vi "main(test) (1).vi"() -> ()   [LabVIEW 2020]
uses:
  stany.ctl
  <vilib>/Analysis/1siggen.llb/Ramp Pattern by Samples.vi
  <vilib>/Utility/file.llb/Write Delimited Spreadsheet (DBL).vi
  lib/VirtualLab.lvlibp/VISASimulator/VISALib.lvlib
  <vilib>/Analysis/NI_AALBase.lvlib
panel:
  in  "save":bool
  out "Connection HP_dvm1":bool
  out "Actual Power [mW]":dbl
  in  "Pmax [mW]":dbl=200.0
  in  "Ib[uA]":dbl(ring) items=["0"=0.0, "100"=0.0001, "200"=0.0002, "300"=0.0003, "400"=0.0004]
  out "Ic=f(Uce)":cluster{dbl[], "Ramp Pattern":dbl[]}(graph)
  out "Ic[A]":dbl
  out "Uce [V]":dbl
  out "Uce=f(Upsu)":cluster{dbl[], "Ramp Pattern":dbl[]}(graph)
  in  "Cancel Button":bool
  out "Progres":u8(slide) scale=0.0..100.0
  in  "stop/resume":bool
  in  "Measure":bool
  in  "Connect":bool
  out "Connection HP_zas":bool
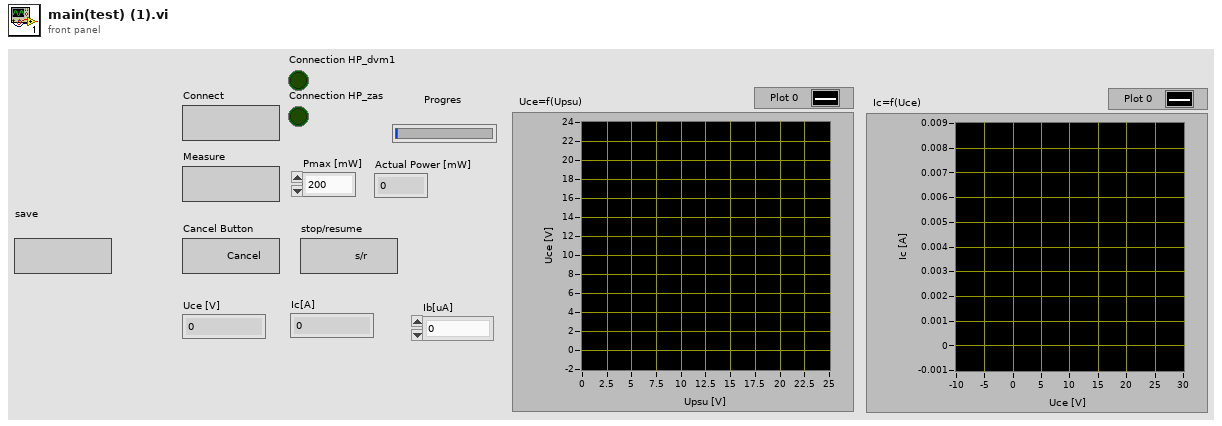
[diagram p1: front panel]
types:
  T1 = cluster{"connecton":bool, "HP_dvm1(DMM reference)":refnum<visa-resource-name>}
  T2 = cluster{"HP_zas (PSU reference)":refnum<visa-resource-name>, "connecton":bool, "Ic":dbl[], "Uce":dbl[]}
  T3 = typedef "stany.ctl" = enum16{"init", "wait", "connect", "measure", "end", "save", "error"}
  T4 = enum8{"Enabled", "Disabled", "Disabled and Grayed Out"}
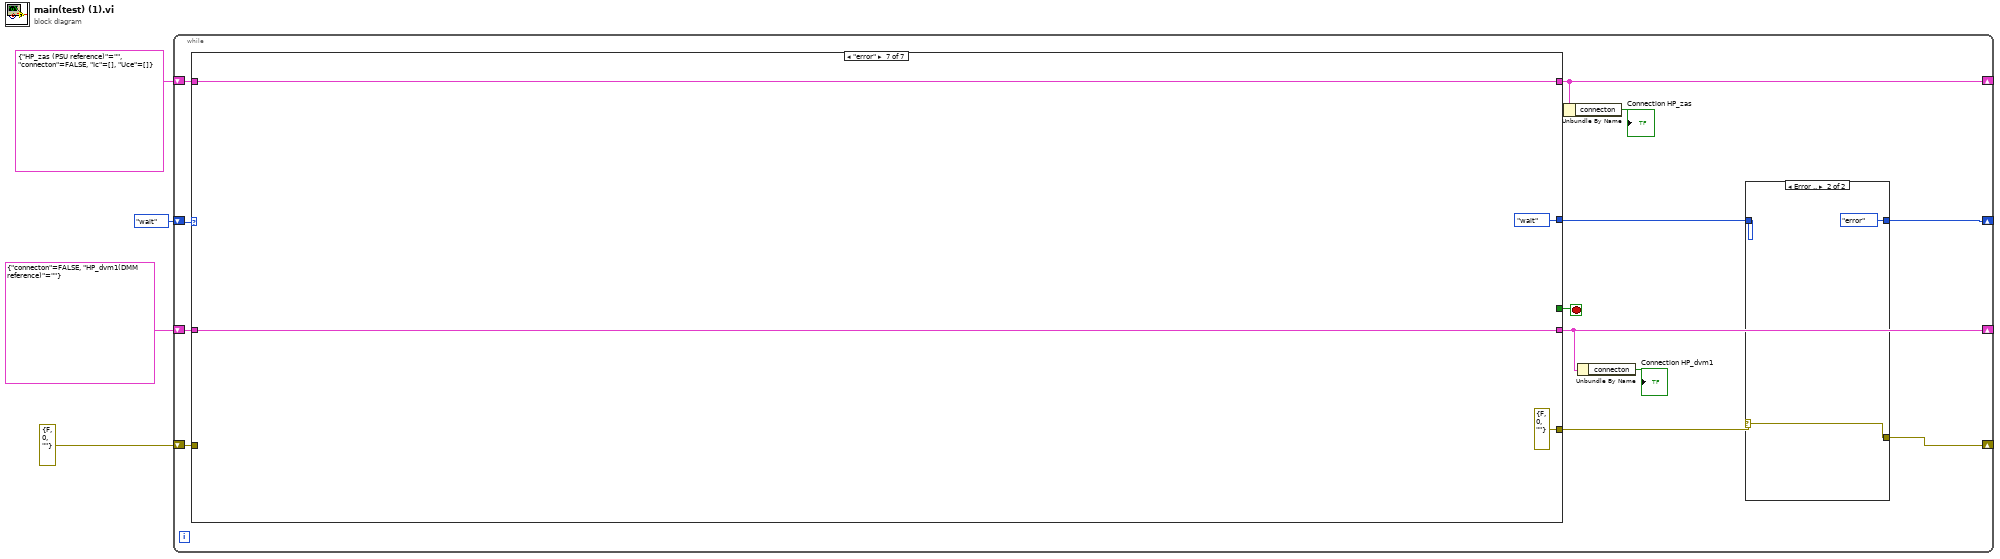
[diagram p0: block diagram]
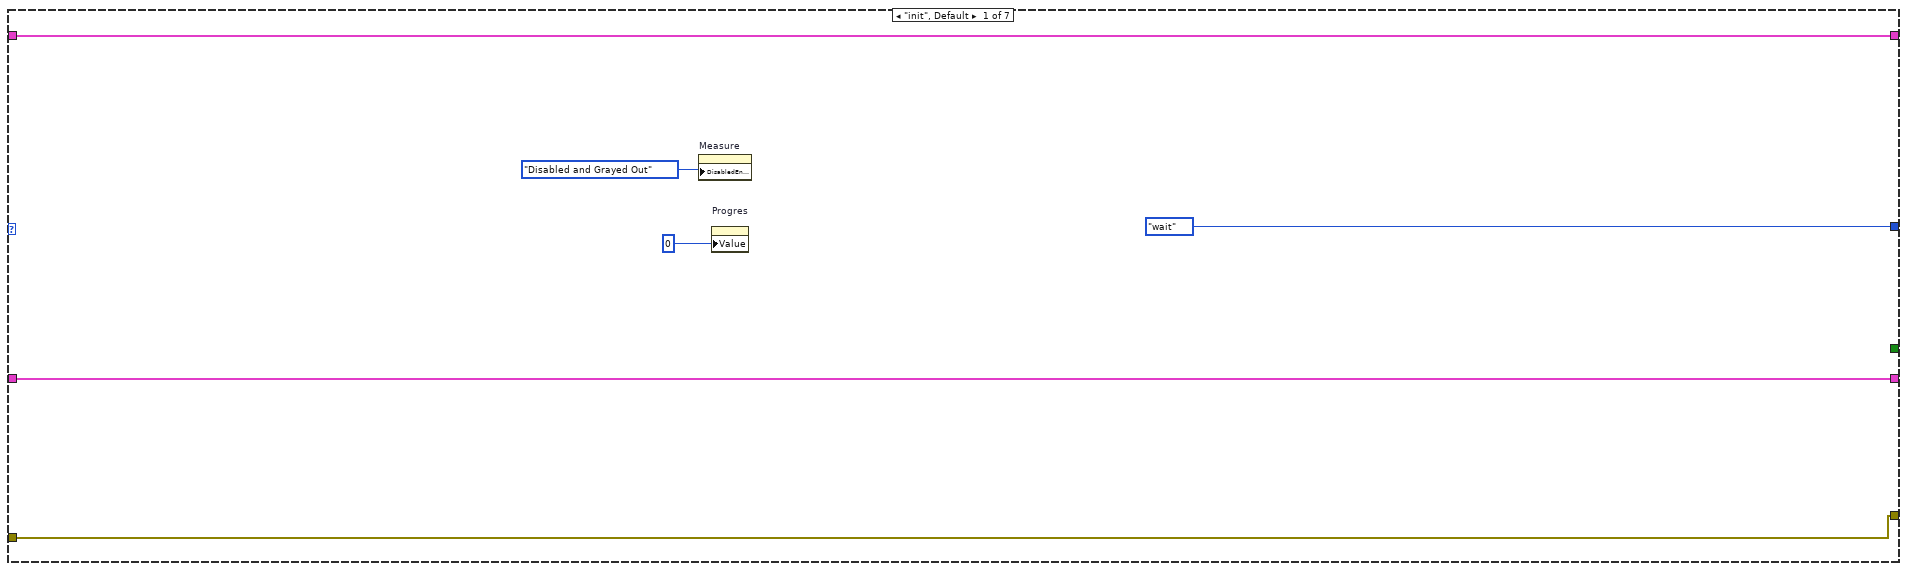
[diagram p3: hidden frame]
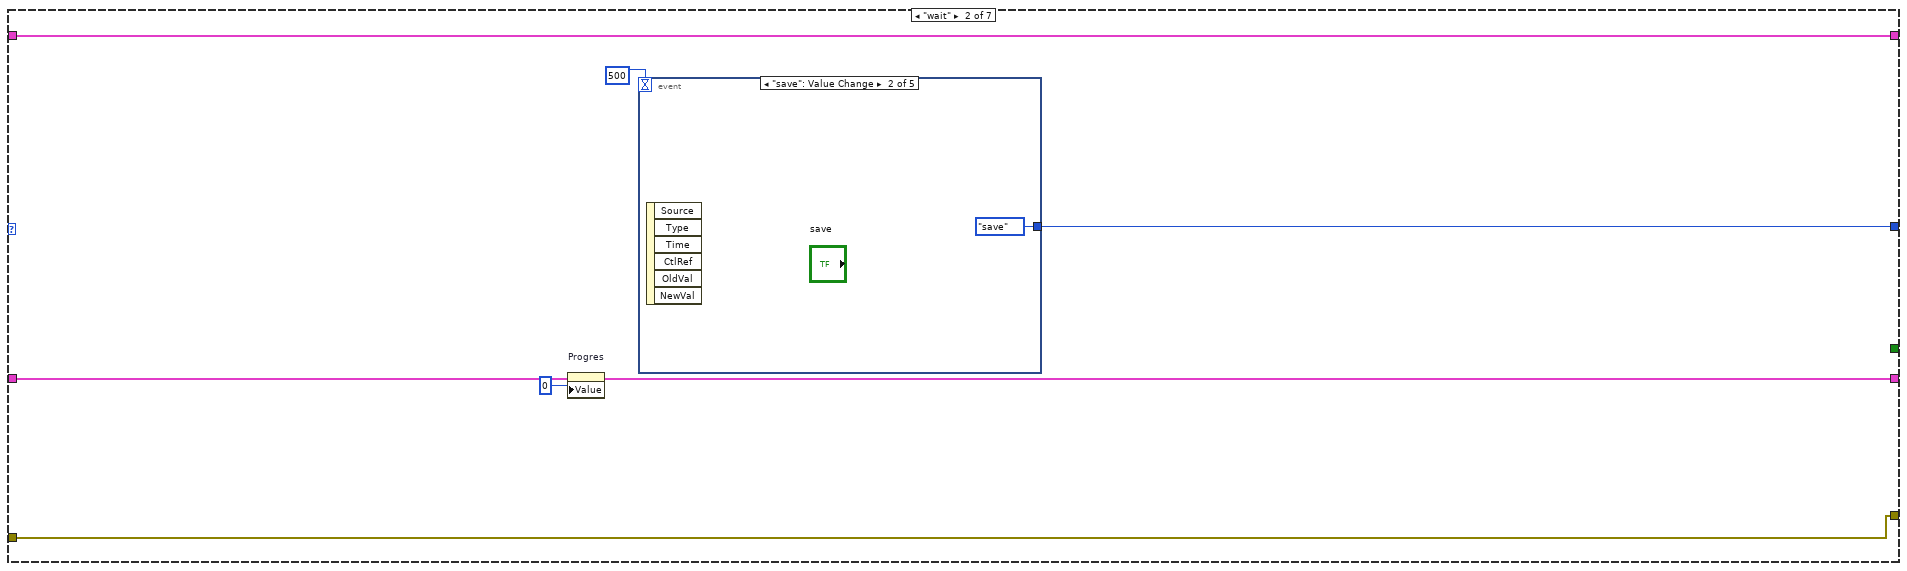
[diagram p4: hidden frame]
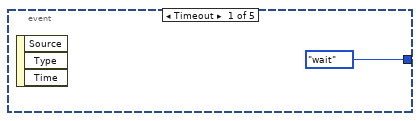
[diagram p5: hidden frame]
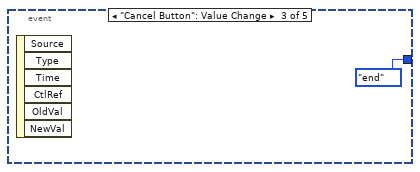
[diagram p6: hidden frame]
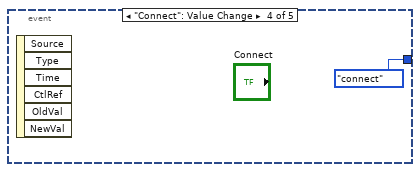
[diagram p7: hidden frame]
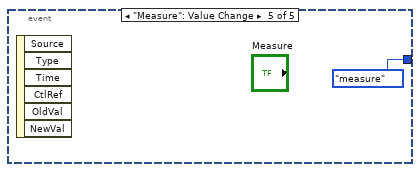
[diagram p8: hidden frame]
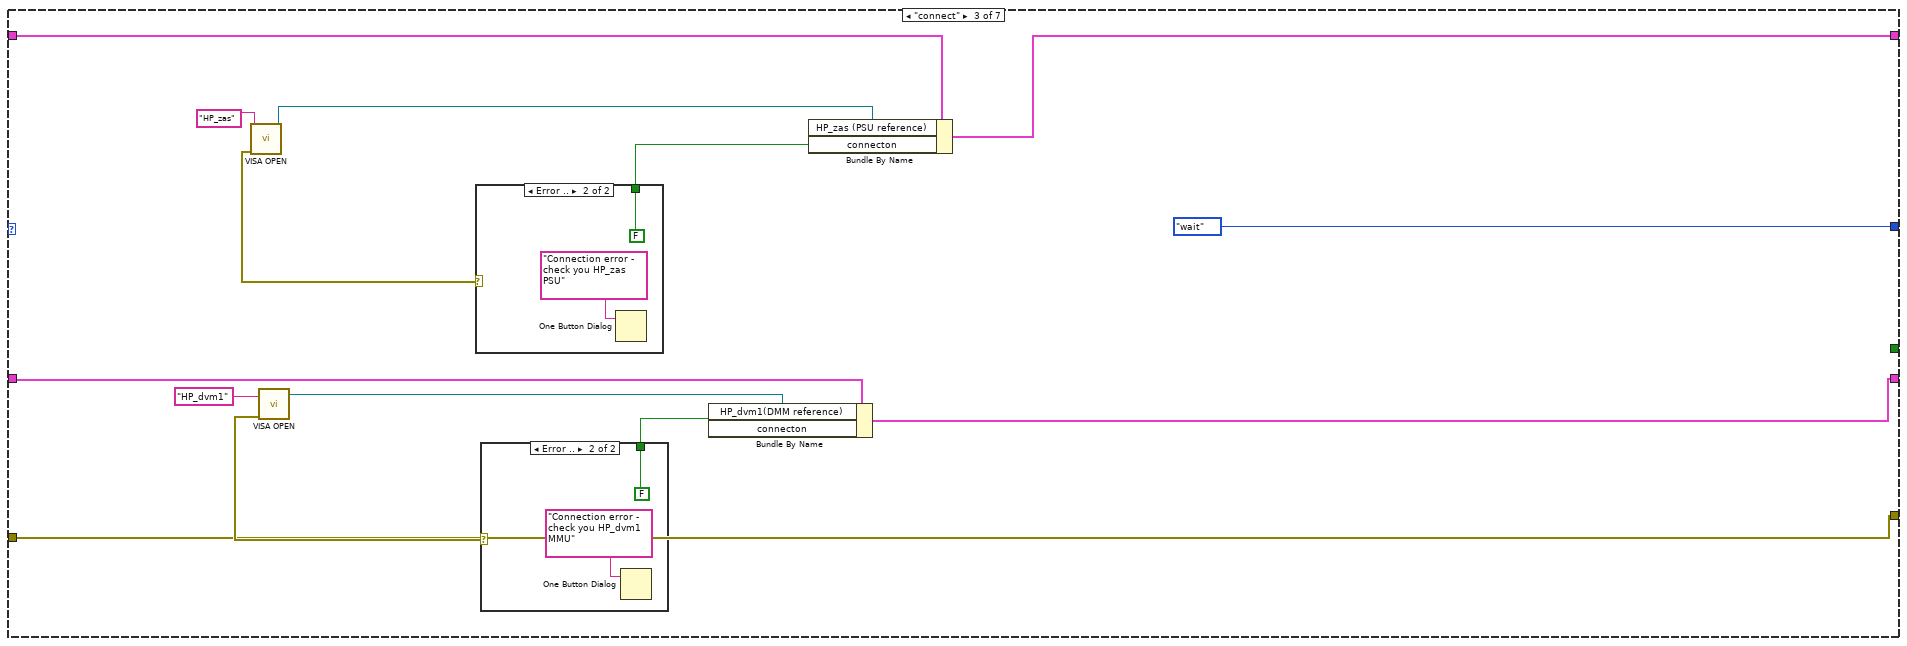
[diagram p9: hidden frame]
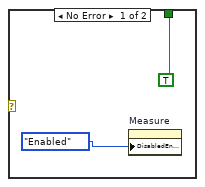
[diagram p10: hidden frame]
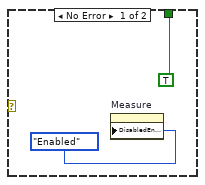
[diagram p11: hidden frame]
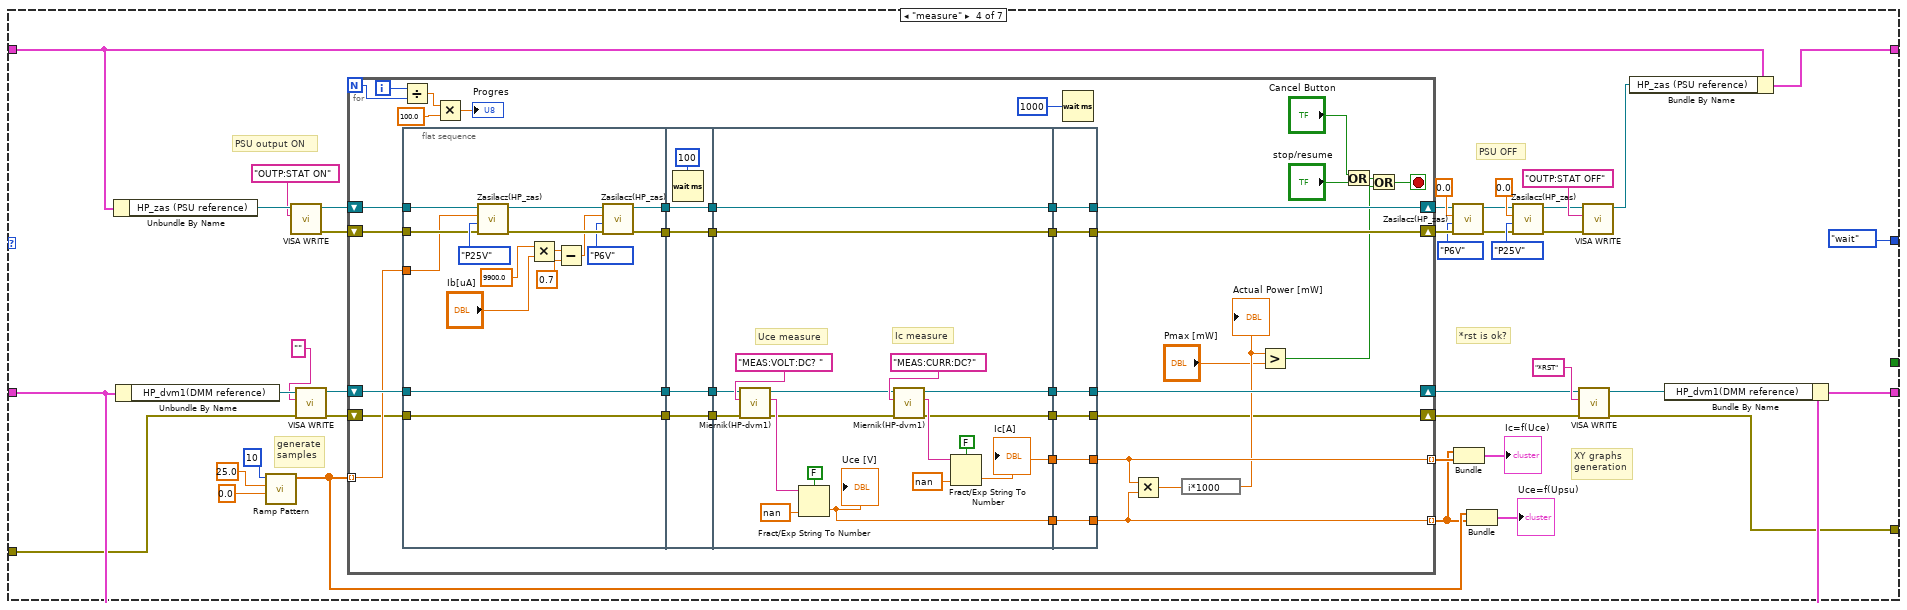
[diagram p12: hidden frame]
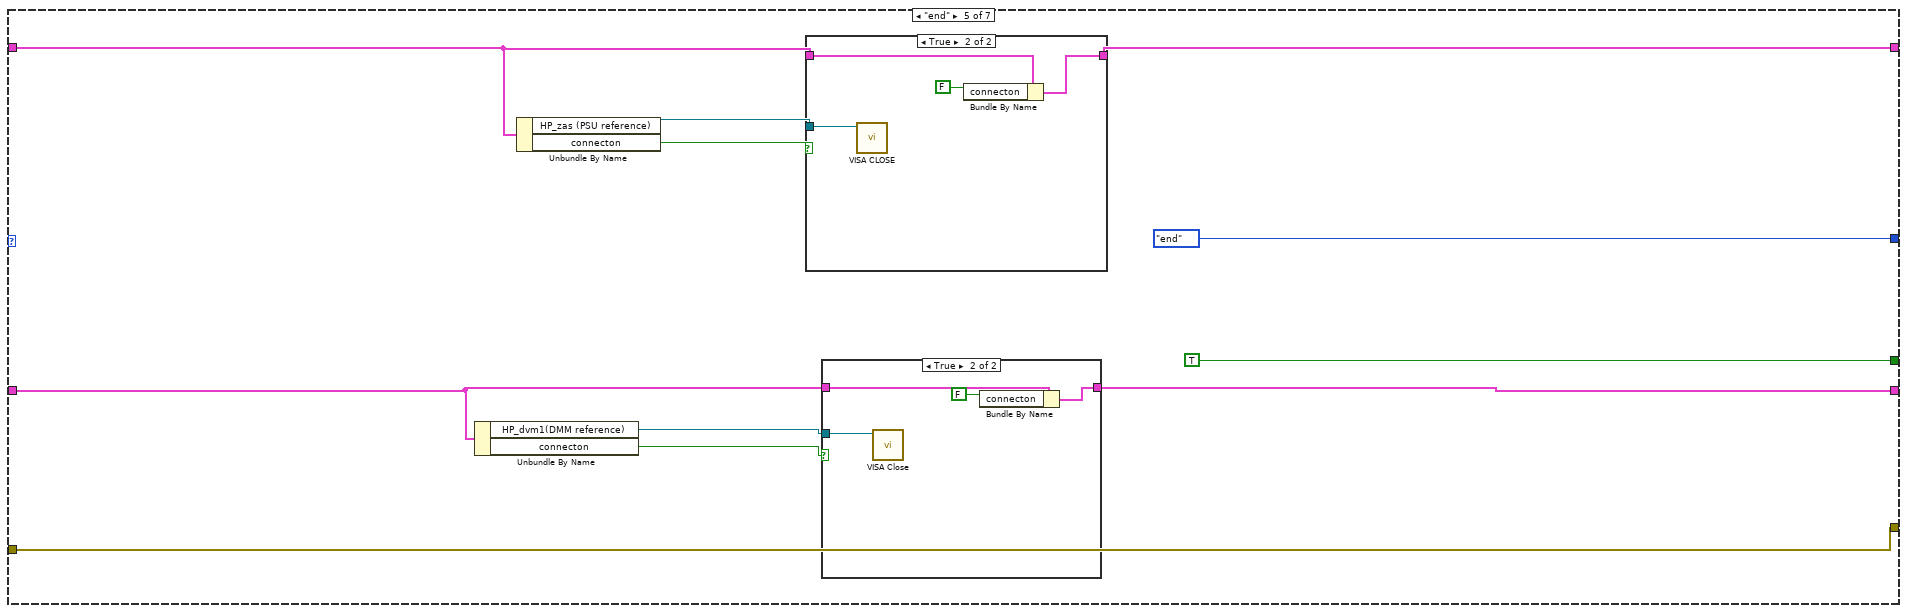
[diagram p13: hidden frame]
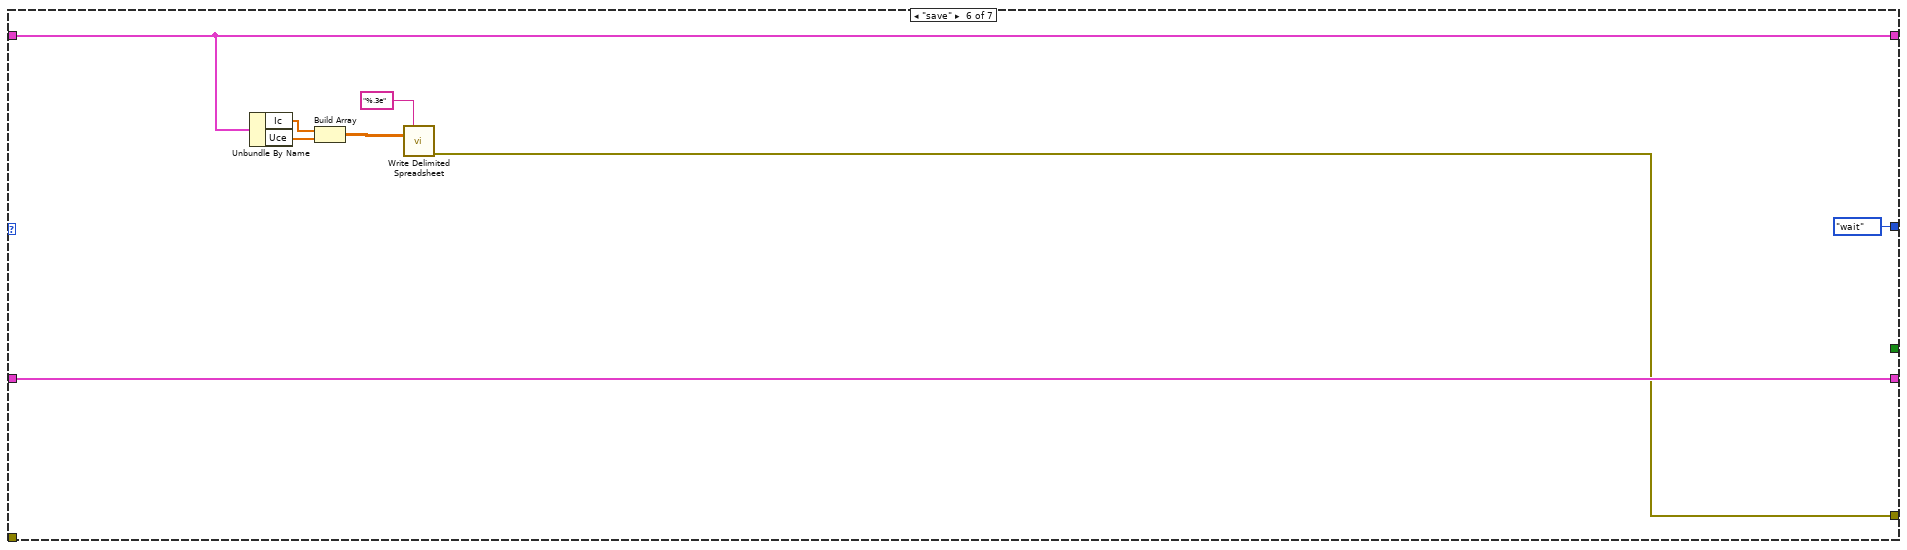
[diagram p16: hidden frame]
diagram:
  n1 = while {
    shift-right: [w5] -> _
    shift-left: stany."wait" -> [w17]
    shift-right: [w13] -> _
    shift-left: T2 {"HP_zas (PSU reference)"="", "connecton"=FALSE, "Ic"=[], "Uce"=[]} -> [w15]
    shift-right: [w10] -> _
    shift-left: T1 {"connecton"=FALSE, "HP_dvm1(DMM reference)"=""} -> [w12]
    shift-right: [w7] -> _
    shift-left: errorcluster {"status"=FALSE, "code"=0, "source"=""} ("error constant") -> [w9]
    stop <- w16 stop-if-true
    n2 = case shown="\"error\"" w17 {
      tunnel: [stany."wait" w32 stany."wait" stany."wait" stany."end" stany."wait" stany."wait"] -> w6
      tunnel: [_ _ _ _ TRUE _ _] -> w16
      tunnel: w15 -> [w25 w31 w47 w98 w190 w210 w216]
      tunnel: [w25 w31 w46 w97 w191 w210 w216] -> w13
      tunnel: w12 -> [w23 w29 w43 w71 w188 w211 w215]
      tunnel: [w23 w29 w42 w72 w185 w211 w215] -> w10
      tunnel: w9 -> [w22 w28 w39 w62 w184 _ _]
      tunnel: [w22 w28 w39 w61 w184 w205 errorcluster {"status"=FALSE, "code"=0, "source"=""} ("error out")] -> w8
      frame "init", Default {
        n3 = property on="Measure" class="Bool"("DisabledEnum"=T4."Disabled and Grayed Out" ("Disabled")) -> ()  [unwired: 2 in, 2 out]
        n4 = property on="Progres" class="Slide (strict)"("Value"=u8 0 ("Progres")) -> ()  [unwired: 2 in, 2 out]
      }
      frame "wait" {
        n5 = property on="Progres" class="Slide (strict)"("Value"=u8 0 ("Progres")) -> ()  [unwired: 2 in, 2 out]
        n6 = event shown="[1] \"save\": Value Change" {
          selector: _ -> [_ _ _ _ _]
          dyn-events: _ -> [_ _ _ _ _]
          timeout: 500 -> [_ _ _ _ _]
          tunnel: [stany."wait" stany."save" stany."end" stany."connect" stany."measure"] -> w32
          event Timeout {
            n7 = event-data() -> ()  [unwired: 1 in, 3 out]
          }
          event "save": Value Change {
            n8 = event-data() -> ()  [unwired: 1 in, 6 out]
          }
          event "Cancel Button": Value Change {
            n9 = event-data() -> ()  [unwired: 1 in, 6 out]
          }
          event "Connect": Value Change {
            n10 = event-data() -> ()  [unwired: 1 in, 6 out]
          }
          event "Measure": Value Change {
            n11 = event-data() -> ()  [unwired: 1 in, 6 out]
          }
        }
      }
      frame "connect" {
        n12 = call "VISA OPEN.vi"("VISA resource name"="HP_zas") -> ("error out"=w50:errorcluster, "VISA resource name out"=w51:refnum<visa-resource-name>)  [unwired: 9 in]
        n13 = call "VISA OPEN.vi"("VISA resource name"="HP_dvm1") -> ("error out"=w40:errorcluster, "VISA resource name out"=w45:refnum<visa-resource-name>)  [unwired: 9 in]
        n14 = case shown="Error .." w50 {
          tunnel: [TRUE FALSE ("connecton")] -> w49
          frame No Error {
            n15 = property on="Measure" class="Bool"("DisabledEnum"=T4."Enabled" ("Disabled")) -> ()  [unwired: 2 in, 2 out]
          }
          frame Error {
            n16 = One Button Dialog(message="Connection error - check you HP_zas PSU") -> ()  [unwired: 1 in, 1 out]
          }
        }
        n17 = case shown="Error .." w40 {
          tunnel: [TRUE FALSE ("connecton")] -> w41
          frame No Error {
            n18 = property on="Measure" class="Bool"("DisabledEnum"=T4."Enabled" ("Disabled")) -> ()  [unwired: 2 in, 2 out]
          }
          frame Error {
            n19 = One Button Dialog(message="Connection error - check you HP_dvm1 MMU") -> ()  [unwired: 1 in, 1 out]
          }
        }
        n20 = Bundle By Name(cluster=w43, "HP_dvm1(DMM reference)"=w45, "connecton"=w41) -> (w42:T1)
        n21 = Bundle By Name(cluster=w47, "HP_zas (PSU reference)"=w51, "connecton"=w49) -> (w46:T2)
      }
      frame "measure" {
        # "*rst is ok?"
        # "XY graphs\ngeneration"
        # "PSU OFF"
        # "PSU output ON"
        # "generate\nsamples"
        n22 = Unbundle By Name(w98) -> ("HP_zas (PSU reference)"=w96:refnum<visa-resource-name>)
        n23 = Unbundle By Name(w71) -> ("HP_dvm1(DMM reference)"=w64:refnum<visa-resource-name>)
        n24 = call-poly <vilib>:"Ramp Pattern.vi"("start"=0.0, "end"=25.0, "samples"=10) -> ("Ramp Pattern"=w80:dbl[])  [unwired: 7 in, 1 out]
        n25 = call "VISA WRITE.vi"("write buffer"="OUTP:STAT ON" ("format string"), "VISA resource name"=w96) -> ("error out"=w84:errorcluster, "VISA resource name out"=w93:refnum<visa-resource-name>)  [unwired: 7 in, 1 out]
        n26 = call "VISA WRITE.vi"("error in (no error)"=w62, "write buffer"="" ("format string"), "VISA resource name"=w64) -> ("error out"=w65:errorcluster, "VISA resource name out"=w66:refnum<visa-resource-name>)  [unwired: 6 in, 1 out]
        n27 = for {
          N -> [w131]
          shift-right: [w127] -> w76
          shift-left: w93 -> [w119]
          tunnel: [w111] -> w73 mode=indexing
          shift-right: [w126] -> w75
          shift-left: w84 -> [w118]
          tunnel: w80 -> [w114] mode=indexing
          tunnel: [w112] -> w81 mode=indexing
          shift-right: [w124] -> w69
          shift-left: w66 -> [w115]
          shift-right: [w104] -> w68
          shift-left: w65 -> [w102]
          i -> [w132]
          stop <- w105 stop-if-true
          n28 = Divide(x=w132, y=w131) -> (x/y=w137:dbl)
          n29 = flat-sequence {
            tunnel: [w147] -> w122
            tunnel: [w148] -> w120
            tunnel: w119 -> [w153]
            tunnel: w118 -> [w152]
            tunnel: [w151] -> w116
            tunnel: w115 -> [w151]
            tunnel: w114 -> [w145]
            tunnel: w102 -> [w139]
            tunnel: [w139] -> w101
            tunnel: [w158] -> w123
            tunnel: w122 -> [w158]
            tunnel: [w157] -> w121
            tunnel: w120 -> [w157]
            tunnel: [w156] -> w117
            tunnel: w116 -> [w156]
            tunnel: w101 -> [w155]
            tunnel: [w155] -> w100
            tunnel: [w171] -> w130
            tunnel: [w172] -> w129
            tunnel: [w173] -> w128
            tunnel: [w163] -> w125
            tunnel: w123 -> [w172]
            tunnel: w121 -> [w171]
            tunnel: w117 -> [w170]
            tunnel: [w162] -> w113
            tunnel: [w161] -> w103
            tunnel: w100 -> [w160]
            tunnel: w130 -> [w182]
            tunnel: w129 -> [w181]
            tunnel: w128 -> [w183]
            tunnel: [w183] -> w111
            tunnel: [w182] -> w127
            tunnel: [w181] -> w126
            tunnel: w125 -> [w180]
            tunnel: [w180] -> w124
            tunnel: w113 -> [w179]
            tunnel: [w179] -> w112
            tunnel: [w178] -> w104
            tunnel: w103 -> [w178]
            frame #0 {
              n30 = call "Zasilacz(HP_zas).vi"("error in (no error)"=w152, "Kanal"=enum16{"P6V", "P25V"}."P25V", "Napiecie"=w145, "VISA Refnum in"=w153) -> ("error out"=w149:errorcluster, "VISA Refnum out"=w150:refnum<visa-resource-name>)  [unwired: 6 in]
              n31 = Multiply(x=9900.0, y="Ib[uA]") -> (x*y=w142:dbl)
              n32 = Subtract(x=w142, y=0.7) -> (x-y=w144:dbl)
              n33 = call "Zasilacz(HP_zas).vi"("error in (no error)"=w149, "Kanal"=enum16{"P6V", "P25V"}."P6V", "Napiecie"=w144, "VISA Refnum in"=w150) -> ("error out"=w147:errorcluster, "VISA Refnum out"=w148:refnum<visa-resource-name>)  [unwired: 6 in]
            }
            frame #1 {
              n34 = Wait (ms)(milliseconds to wait=u32 100) -> ()  [unwired: 1 out]
            }
            frame #2 {
              # "Ic measure"
              # "Uce measure"
              n35 = call "Miernik(HP-dvm1).vi"("error in (no error)"=w160, "write buffer"="MEAS:VOLT:DC? ", "VISA Refnum in"=w170) -> ("error out"=w165:errorcluster, "read buffer"=w177:string, "VISA Refnum out"=w164:refnum<visa-resource-name>)  [unwired: 6 in]
              n36 = Fract/Exp String To Number(use system decimal point (T)=FALSE, string=w177, default (0 dbl)=nan) -> (number=w173:dbl)  [unwired: 1 in, 1 out]
              "Uce [V]" <- w173
              n37 = call "Miernik(HP-dvm1).vi"("error in (no error)"=w165, "write buffer"="MEAS:CURR:DC?", "VISA Refnum in"=w164) -> ("error out"=w161:errorcluster, "read buffer"=w169:string, "VISA Refnum out"=w163:refnum<visa-resource-name>)  [unwired: 6 in]
              n38 = Fract/Exp String To Number(use system decimal point (T)=FALSE, string=w169, default (0 dbl)=nan) -> (number=w162:dbl)  [unwired: 1 in, 1 out]
              "Ic[A]" <- w162
            }
            frame #3 {
            }
          }
          n39 = Multiply(x=w137, y=100.0) -> (x*y=→"Progres":dbl)
          n40 = Wait (ms)(milliseconds to wait=u32 1000) -> ()  [unwired: 1 out]
          n41 = Multiply(x=w112, y=w111) -> (x*y=w110:dbl)
          n42 = expression code="i*1000"(w110) -> (w109:dbl)
          "Actual Power [mW]" <- w109
          n43 = Greater?(x=w109, y="Pmax [mW]") -> (0:w106:bool)
          n44 = Or(x="Cancel Button", y="stop/resume") -> (x .or. y?=w107:bool)
          n45 = Or(x=w107, y=w106) -> (x .or. y?=w105:bool)
        }
        n46 = call "Zasilacz(HP_zas).vi"("error in (no error)"=w75, "Kanal"=enum16{"P6V", "P25V"}."P6V", "Napiecie"=0.0 ("Napiecie 2"), "VISA Refnum in"=w76) -> ("error out"=w78:errorcluster, "VISA Refnum out"=w77:refnum<visa-resource-name>)  [unwired: 6 in]
        n47 = Bundle(w73, w81) -> (→"Ic=f(Uce)":cluster{dbl[], dbl[]})  [unwired: 1 in]
        n48 = Bundle("Ramp Pattern"=w80, w73) -> (→"Uce=f(Upsu)":cluster{"Ramp Pattern":dbl[], dbl[]})  [unwired: 1 in]
        n49 = call "Zasilacz(HP_zas).vi"("error in (no error)"=w78, "Kanal"=enum16{"P6V", "P25V"}."P25V", "Napiecie"=0.0 ("Napiecie 2"), "VISA Refnum in"=w77) -> ("error out"=w85:errorcluster, "VISA Refnum out"=w86:refnum<visa-resource-name>)  [unwired: 6 in]
        n50 = call "VISA WRITE.vi"("error in (no error)"=w68, "write buffer"="*RST" ("format string"), "VISA resource name"=w69) -> ("error out"=w61:errorcluster, "VISA resource name out"=w67:refnum<visa-resource-name>)  [unwired: 6 in, 1 out]
        n51 = call "VISA WRITE.vi"("error in (no error)"=w85, "write buffer"="OUTP:STAT OFF" ("format string"), "VISA resource name"=w86) -> ("VISA resource name out"=w92:refnum<visa-resource-name>)  [unwired: 6 in, 2 out]
        n52 = Bundle By Name(cluster=w98, "HP_zas (PSU reference)"=w92) -> (w97:T2)
        n53 = Bundle By Name(cluster=w71, "HP_dvm1(DMM reference)"=w67) -> (w72:T1)
      }
      frame "end" {
        n54 = Unbundle By Name(w188) -> ("HP_dvm1(DMM reference)"=w186:refnum<visa-resource-name>, "connecton"=w187:bool)
        n55 = Unbundle By Name(w190) -> ("HP_zas (PSU reference)"=w192:refnum<visa-resource-name>, "connecton"=w189:bool)
        n56 = case shown="True" w189 {
          tunnel: w192 -> [_ w204]
          tunnel: w190 -> [w200 w203]
          tunnel: [w200 w201] -> w191
          frame False {
          }
          frame True {
            n57 = call "VISA CLOSE.vi"("VISA resource name"=w204) -> ()  [unwired: 10 in, 1 out]
            n58 = Bundle By Name(cluster=w203, "connecton"=FALSE) -> (w201:T2)
          }
        }
        n59 = case shown="True" w187 {
          tunnel: w186 -> [_ w199]
          tunnel: w188 -> [w195 w198]
          tunnel: [w195 w196] -> w185
          frame False {
          }
          frame True {
            n60 = call "VISA Close.vi"("VISA resource name"=w199) -> ()  [unwired: 10 in, 1 out]
            n61 = Bundle By Name(cluster=w198, "connecton"=FALSE) -> (w196:T1)
          }
        }
      }
      frame "save" {
        n62 = Unbundle By Name(w210) -> ("Ic"=w209:dbl[], "Uce"=w208:dbl[])
        n63 = Build Array(w209, w208) -> (w207:dbl[][])
        n64 = call-poly <vilib>:"Write Delimited Spreadsheet.vi"("format (%.3f)"="%.3e", "2D data"=w207) -> ("error out"=w205:errorcluster)  [unwired: 12 in, 1 out]
      }
      frame "error" {
      }
    }
    n65 = Unbundle By Name(w13) -> ("connecton"=→"Connection HP_zas":bool)
    n66 = Unbundle By Name(w10) -> ("connecton"=→"Connection HP_dvm1":bool)
    n67 = case shown="Error .." w8 {
      selector: w8 -> [w19 w20]
      tunnel: [w19 w20] -> w7
      tunnel: w6 -> [w18 _]
      tunnel: [w18 stany."error"] -> w5
      frame No Error {
      }
      frame Error {
      }
    }
  }
